vi "int_string_noSpace.vi"(11 "Numeric":dbl) -> (3 "int string out":string)   [LabVIEW 2016]
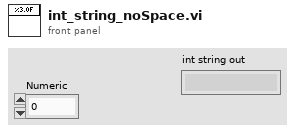
[diagram p1: front panel]
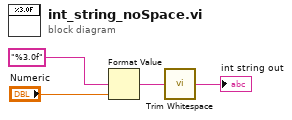
[diagram p0: block diagram]
diagram:
  n1 = Format Value(format string="%3.0f", value (0)="Numeric") -> (output string=w2:string)  [unwired: 1 in]
  n2 = call <vilib>:"Trim Whitespace.vi"("string"=w2) -> ("trimmed string"=→"int string out":string)  [unwired: 1 in]
